vi "Write.vi"(8 "error in (no error)":errorcluster, 11 "Hardware Resources in":T1) -> (0 "error out":errorcluster, 3 "Hardware Resources out":T1)   [LabVIEW 2018, in "DAQ.lvlib"]
doc: "Perform the acquisition. Replace the contents of this diagram with calls to acquisition hardware."
uses:
  DAQ.lvlib
  Hardware Configuration.ctl
  Acquisition/Task Cluster.ctl
  <vilib>/DAQmx/write.llb/DAQmx Write (Analog DBL 1Chan 1Samp).vi
  <vilib>/DAQmx/miscellaneous.llb/DAQmx Fill In Error Info.vi
  <resource>/objmgr/daqmx.rc
  DAQ/DAQ Write.lvlib
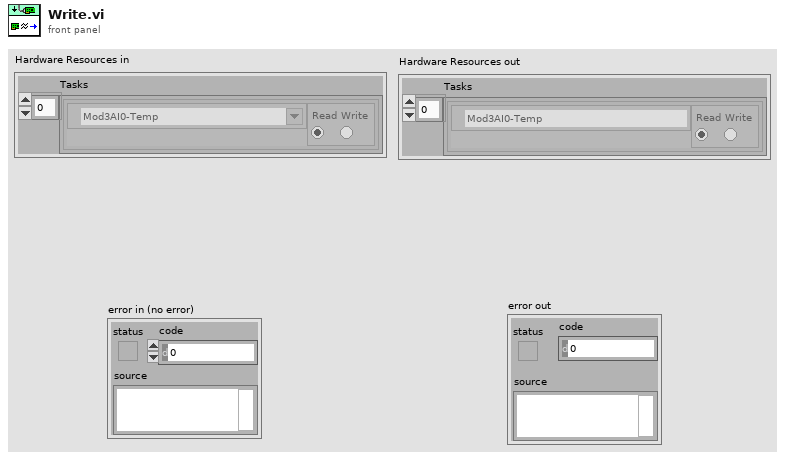
[diagram p1: front panel]
types:
  T1 = typedef "DAQ.lvlib/DAQ Write.lvlib/Hardware Configuration.ctl" = cluster{"Tasks":T2[]}
  T2 = typedef "Task Cluster.ctl" = cluster{"DAQmx Task":refnum<k21>, "Read-Write Radio":enum32{"Read", "Write"}}
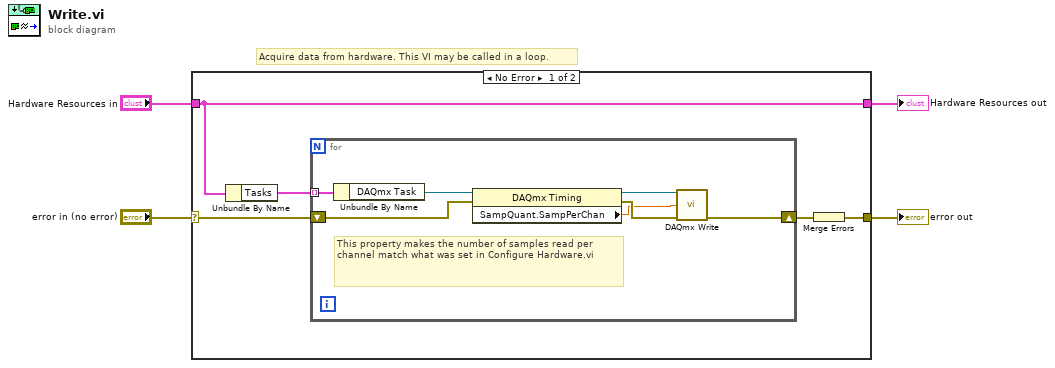
[diagram p0: block diagram]
diagram:
  # "Acquire data from hardware. This VI may be called in a loop."
  n1 = case shown="No Error" "error in (no error)" {
    selector: "error in (no error)" -> [w5 w17]
    tunnel: [w9 w17] -> w3
    tunnel: "Hardware Resources in" -> [w8 w18]
    tunnel: [w8 w18] -> w1
    frame No Error {
      n2 = Unbundle By Name(w8) -> ("Tasks"=w6:T2[])
      n3 = for {
        tunnel: w6 -> [w15] mode=indexing
        shift-right: [w16] -> w7
        shift-left: w5 -> [w13]
        # "This property makes the number of samples read per channel match what was set in Configure Hardware.vi"
        n4 = Unbundle By Name(w15) -> ("DAQmx Task"=w11:refnum<k21>)
        n5 = property class="DAQmx Timing"(reference=w11, error in=w13) -> (reference out=w14:refnum<k21>, error out=w12:errorcluster, "SampQuant.SampPerChan"=w10:dbl)
        n6 = call-poly <vilib>:"DAQmx Write.vi"("task/channels in"=w14, "data"=w10, "error in"=w12) -> ("error out"=w16:errorcluster)  [unwired: 10 in, 2 out]
      }
      n7 = Merge Errors(w7) -> (w9:errorcluster)
    }
    frame Error {
    }
  }
  "Hardware Resources out" <- w1
  "error out" <- w3
